vi "TCP read until EOL.vi"(3 "error in (no error)":errorcluster, 4 "Read limit (10240)":u32=10240, 5 "Timeout (5000 msec)":i32=5000, 6 "connection ID":refnum<k5>) -> (0 "error out":errorcluster, 1 "Final string":string, 2 "Error":bool)   [LabVIEW 2009]
doc: "A subroutine that reads from an open TCP connection, one byte at a time, until it gets a newline chararacter. It then returns the string up to the newline.\n\nDesigned to read line-delimited commands from another process. This is re-entrant and called from many other vis. \n\nNote also that it now accepts either newline or carriage return as end-of-line, but the DOS convention of CR+LF will not work correctly."
panel:
  out "Number of reads":u32
  in  "Read size (1 byte)":u32=1
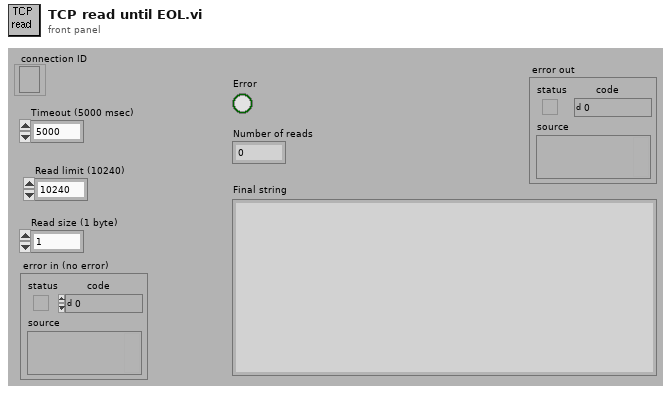
[diagram p1: front panel]
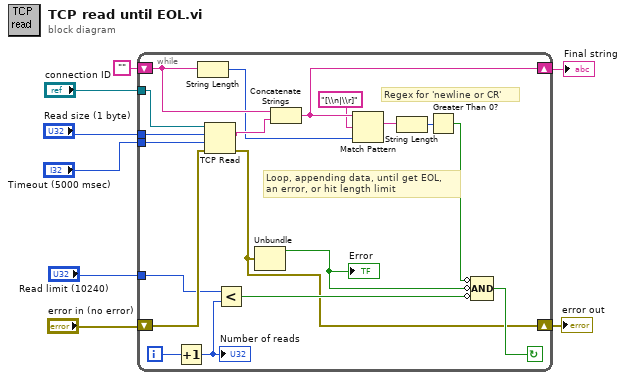
[diagram p0: block diagram]
diagram:
  n1 = while {
    shift-right: [w21] -> w4
    shift-left: "" -> [w13]
    shift-right: [w11] -> w2
    shift-left: "error in (no error)" -> [w27]
    tunnel: "Timeout (5000 msec)" -> [w26]
    tunnel: "Read size (1 byte)" -> [w25]
    tunnel: "connection ID" -> [w24]
    tunnel: "Read limit (10240)" -> [w17]
    i -> [w22]
    stop <- w15 continue-if-true
    # "Regex for 'newline or CR'"
    # "Loop, appending data, until get EOL,\nan error, or hit length limit"
    n2 = Increment(x=w22) -> (x+1=w18:i32)
    "Number of reads" <- w18
    n3 = String Length(string=w13) -> (length=w12:i32)
    n4 = TCP Read(connection ID=w24, bytes to read=w25, error in (no error)=w27, 9:w26) -> (data out=w23:string, error out=w11:errorcluster)  [unwired: 2 out]
    n5 = Less?(x=w17, y=w18) -> (x < y?=w16:bool)
    n6 = Unbundle(w11) -> ("status"=w10:bool)  [unwired: 2 out]
    "Error" <- w10
    n7 = Concatenate Strings(w13, w23) -> (w21:string)
    n8 = Match Pattern(string=w21, regular expression="[\\n|\\r]", offset (0)=w12) -> (match substring=w14:string)  [unwired: 3 out]
    n9 = String Length(string=w14) -> (length=w20:i32)
    n10 = Greater Than 0?(x=w20) -> (x > 0?=w19:bool)
    n11 = Compound Arithmetic op=AND(invert w19, invert w10, invert w16) -> (w15:bool)
  }
  "Final string" <- w4
  "error out" <- w2
